vi "Insert Created.vi"(8 "Queue":refnum<data-value>, 9 "Queue Self Alias":string, 10 "Queue Mailbox in":refnum<data-value>) -> (0 "error out":errorcluster, 2 "Queue Mailbox out":refnum<data-value>)   [LabVIEW 2021, in "jettl.lvlib"]
uses:
  jettl.lvlib
  Queue Mailbox/Queue Mailbox.lvclass
  Msg Strategy/Msg Strategy.lvclass
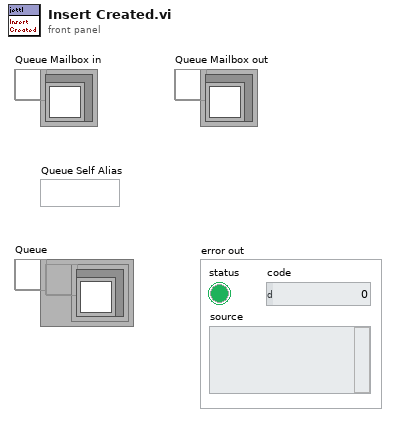
[diagram p1: front panel]
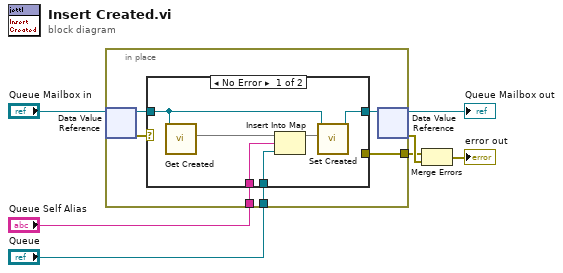
[diagram p0: block diagram]
diagram:
  n1 = in-place {
    in-place-border: [w13] -> w3
    in-place-border: "Queue Self Alias" -> [w10]
    in-place-border: "Queue" -> [w8]
    n2 = in-place-dvr #1("Queue Mailbox in") -> (w11:refnum<class "Queue Mailbox.lvclass">, w12:errorcluster)
    n3 = case shown="No Error" w12 {
      selector: w12 -> [_ w21]
      tunnel: w11 -> [w16 w20]
      tunnel: [_ w21] -> w13
      tunnel: w10 -> [w18 _]
      tunnel: [w15 w20] -> w9
      tunnel: w8 -> [w14 _]
      frame No Error {
        n4 = call "Get Created.vi"("Queue Mailbox in"=w16) -> ("Created"=w19:map{string, refnum<data-value>})  [unwired: 10 in]
        n5 = Insert Into Map(map in=w19, key=w18, value=w14) -> (map out=w17:map{string, refnum<data-value>})  [unwired: 2 out]
        n6 = call "Set Created.vi"("Created"=w17, "Queue Mailbox in"=w16) -> ("Queue Mailbox out"=w15:refnum<class "Queue Mailbox.lvclass">)  [unwired: 9 in]
      }
      frame Error {
      }
    }
    n7 = in-place-dvr #1(w9) -> (→"Queue Mailbox out":refnum<data-value>, w4:errorcluster)
  }
  n8 = Merge Errors(w3, w4) -> (→"error out":errorcluster)
